vi "createFilepath.vi"(1 "filename":string, 2 "path":path) -> (0 "file path":path)   [LabVIEW 2015]
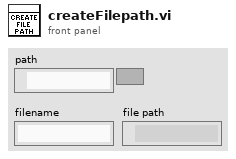
[diagram p1: front panel]
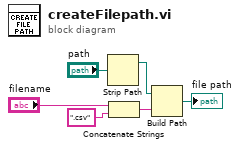
[diagram p0: block diagram]
diagram:
  n1 = Strip Path(path="path") -> (stripped path=w3:path)  [unwired: 1 out]
  n2 = Concatenate Strings("filename", ".csv" ("string")) -> (w4:string)
  n3 = Build Path(base path=w3, name or relative path=w4) -> (appended path=→"file path":path)
